vi "Init.vi"(5 "Stop User Event in":refnum<user-event>, 7 "Ref FP in":refnum<vi>, 8 "error in (no error)":errorcluster, 9 "Period (ms) in":i64=15, 11 "Input Device in":refnum<class "Input Device.lvclass">) -> (0 "error out":errorcluster, 3 "Input Device out":refnum<class "Input Device.lvclass">)   [LabVIEW 2024, in "Input Device.lvclass"]
doc: "MIT Licence\nCopyright (c) 2024 David Grollier"
uses:
  Input Device.lvclass
  Input Device.lvclass/Input Device.ctl
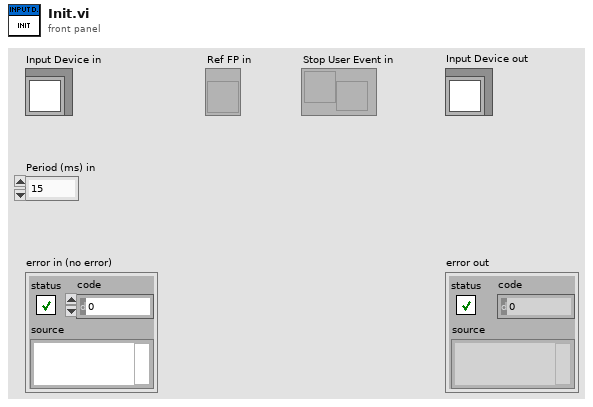
[diagram p1: front panel]
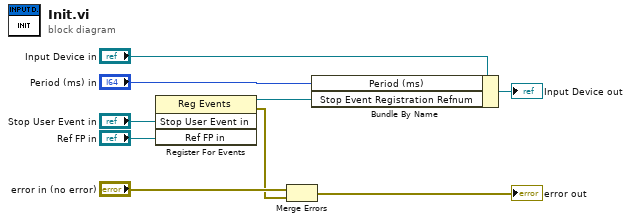
[diagram p0: block diagram]
diagram:
  n1 = register-events("Stop User Event in", "Ref FP in") -> (reference out=w5:refnum<event-registration>, error out=w3:errorcluster)  [unwired: 2 in]
  n2 = Merge Errors("error in (no error)", w3) -> (→"error out":errorcluster)
  n3 = Bundle By Name(cluster="Input Device in", "Period (ms)"="Period (ms) in", "Stop Event Registration Refnum"=w5) -> (→"Input Device out":refnum<class "Input Device.lvclass">)
